vi "dataset.label_at.vi"(8 "error in":errorcluster, 11 "Dataset in":refnum<class "Dataset.lvclass">) -> (0 "error out":errorcluster, 3 "Dataset out":refnum<class "Dataset.lvclass">)   [LabVIEW 2020, in "Dataset.lvclass"]
doc: "Returns the label at the given index."
uses:
  Dataset.lvclass
  Dataset.lvclass/Dataset.ctl
  client.lvlib
panel:
  out "out_needed out":u32
  out "label":string
  in  "index":i32
  in  "buf":string
  in  "cap":u32
  in  "out_needed":u32
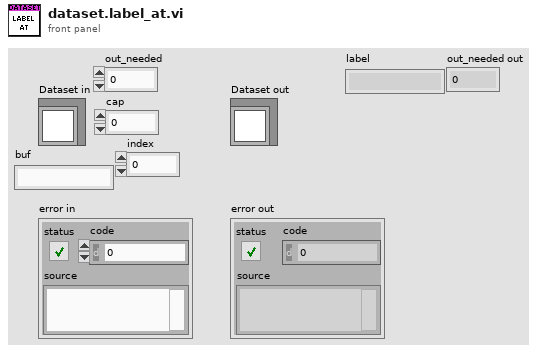
[diagram p1: front panel]
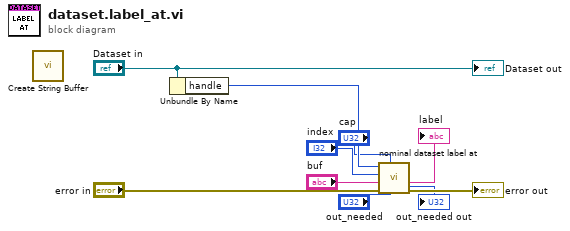
[diagram p0: block diagram]
diagram:
  n1 = call "Create String Buffer.vi"() -> ()  [unwired: 9 in, 3 out]
  n2 = Unbundle By Name("Dataset in") -> ("handle"=w8:i32)
  n3 = call "nominal dataset label at.vi"("out_needed"="out_needed", "cap"="cap", "error in (no error)"="error in", "buf"="buf", "index"="index", "dataset"=w8) -> ("error out"=→"error out":errorcluster, "buf out"=→"label":string, "out_needed out"=→"out_needed out":u32)  [unwired: 2 in, 1 out]
  "Dataset out" <- "Dataset in"
